vi "XY Graph Is Plot Valid.vi"(2 "Plot":T1) -> (7 "Is Valid Plot?":bool)   [LabVIEW 2021, in "XY Graph Add-Ons.lvlib"]
uses:
  XY Graph Add-Ons.lvlib
  XY Graph Plot Data.ctl
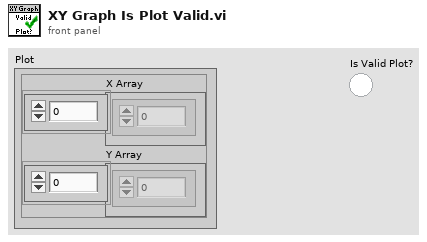
[diagram p1: front panel]
types:
  T1 = typedef "XY Graph Add-Ons.lvlib/XY Graph Plot Data.ctl" = cluster{"X Array":dbl[], "Y Array":dbl[]}
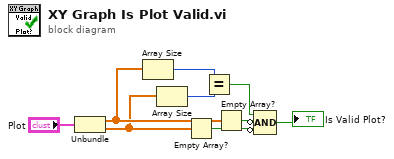
[diagram p0: block diagram]
diagram:
  n1 = Unbundle("Plot") -> ("X Array"=w6:dbl[], "Y Array"=w5:dbl[])
  n2 = Array Size(array=w6) -> (size(s)=w4:i32)
  n3 = Array Size(array=w5) -> (size(s)=w3:i32)
  n4 = Empty Array?(array=w5) -> (empty?=w8:bool)
  n5 = Equal?(x=w4, y=w3) -> (x = y?=w2:bool)
  n6 = Empty Array?(array=w6) -> (empty?=w9:bool)
  n7 = Compound Arithmetic op=AND(w2, invert w9, invert w8) -> (→"Is Valid Plot?":bool)
